vi "Create Tag Loop.vi"(8 "error in (no error)":errorcluster, 9 "Tag Category":string, 10 "data type":T1(ring), 11 "Tag Name":string) -> (0 "error out":errorcluster)   [LabVIEW 2018, in "Support Library.lvlib"]
uses:
  Support Library.lvlib
  Tag VIs/Tag FGV Operation Enum.ctl
  Shared Variables/Dynamic Shared Variables.lvlib
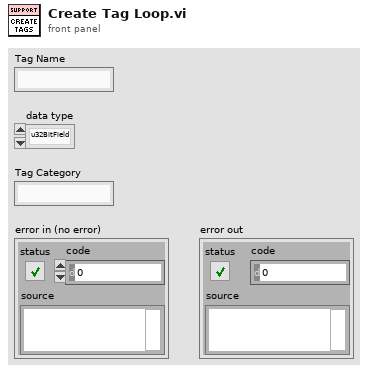
[diagram p1: front panel]
types:
  T1 = enum32{"u32BitField", "bool", "double", "string", "int8", "uint8", "int16", "uint16", "int32", "uint32", "int64", "uint64", "single", "double waveform", "int16 waveform", "array of boolean", "array of int8", "array of uint8", "array of int16", "array of uint16", "array of int32", "array of uint32", "array of int64", "array of uint64", "array of single", "array of double", "array of double waveform", "array of int16 waveform", "array of string", "variant", "timestamp", "fixed point", "custom"}
  T2 = typedef "Tag FGV Operation Enum.ctl" = enum16{"Init", "Set Notification Queue", "Create Tag", "Commit", "Write Tag (Numeric)", "Write Tag (Boolean)", "Read All Tags", "Read One Tag", "Delete Tag Category", "Set Alarm Parameters (Numeric)", "Set Alarm Parameters (Boolean)", "Enable All Alarms", "Disable All Alarms", "Delete All Tags", "Read Alarms", "Ack Alarm", "Read Alarm Parameters (Numeric)", "Read Alarm Parameters (Boolean)"}
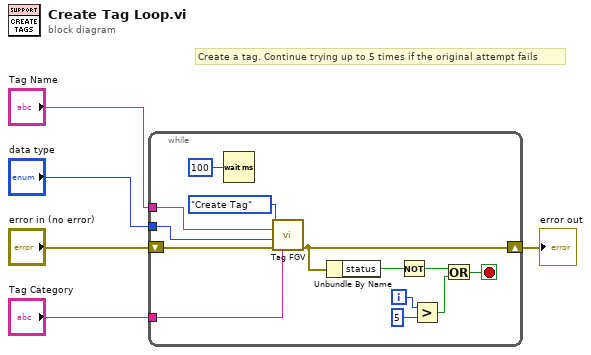
[diagram p0: block diagram]
diagram:
  # "Create a tag. Continue trying up to 5 times if the original attempt fails"
  n1 = while {
    tunnel: "Tag Name" -> [w10]
    tunnel: "Tag Category" -> [w6]
    shift-right: [w7] -> w3
    shift-left: "error in (no error)" -> [w8]
    tunnel: "data type" -> [w9]
    i -> [w14]
    stop <- w12 stop-if-true
    n2 = Wait (ms)(milliseconds to wait=u32 100) -> ()  [unwired: 1 out]
    n3 = call "Tag FGV.vi"("Operation"=Tag_FGV_Operation_Enum."Create Tag", "Tag Name"=w10, "Data"=w9, "error in (no error)"=w8, "Tag Category"=w6) -> ("error out"=w7:errorcluster)  [unwired: 3 in, 7 out]
    n4 = Unbundle By Name(w7) -> ("status"=w18:bool)
    n5 = Not(x=w18) -> (.not. x?=w16:bool)
    n6 = Greater?(x=w14, y=5 ("x")) -> (0:w13:bool)
    n7 = Or(x=w16, y=w13) -> (x .or. y?=w12:bool)
  }
  "error out" <- w3
